vi "Man Simulation V2.vi"() -> ()   [LabVIEW 2020]
panel:
  out "J in 1 NS pair with gap":dbl
  out "Energy (wh/m3) / 1 NS pari with gap":dbl
  out "Energy Density  WH/m3":dbl
  in  "Energy Density  WH/Lit":dbl
  out "1 NS Pair Energy / Volume":dbl
  out "1 NS Pair Energy / mass":dbl
  out "Chip Energy Wh":dbl
  out "WH/Lit":dbl
  out "WH/m3":dbl
  out "WH/Kg":dbl
  out "Chip Energy / Volume":dbl
  out "Chip Energy /Mass":dbl
  out "Mass of a Chip":dbl
  out "Volume of a Chip":dbl
  out "Mass NS Pair with Gap":dbl
  out "Volume NS Pair With Gap":dbl
  out "Volume Gap":dbl
  out "Mass Gap":dbl
  out "Delta Temp Change \nDielectric Gap":dbl
  out "Dielectric Thickness  \nGap":dbl
  out "Mass Dielectric \nGap":dbl
  out "Volume Dielectric \nGap":dbl
  out "Delta Temp Change\n SiO2 Gap":dbl
  out "Mass SiO2 Gap":dbl
  out "Sio2 Thickness Gap":dbl
  out "Volume SiO2 Gap":dbl
  out "Volume Si Gap":dbl
  out "Silicon Thickness Gap":dbl
  out "Mass Si Gap":dbl
  out "Delta Temp Change\n Si Gap":dbl
  out "Area B/W NS":dbl
  out "Vol 2 NS":dbl
  out "Mass 2 NS":dbl
  out "Mass 1 NS":dbl
  out "Volume 1 NS":dbl
  out "SiO2 Specfic Heat Capacity 2":dbl
  out "SilO2 Density 2":dbl
  out "Delta Temp Change SiO2 2":dbl
  out "Mass SiO2 2":dbl
  out "Volume SiO2 2":dbl
  out "Dielectric Specfic Heat Capacity":dbl
  out "Dielectric Density":dbl
  out "CNT Specfic Heat Capacity":dbl
  out "CNT Density":dbl
  out "Fe Specfic Heat Capacity":dbl
  out "Fe Density":dbl
  out "Al Specfic Heat Capacity":dbl
  out "Al Density":dbl
  out "Al2O3 Specfic Heat Capacity":dbl
  out "Al2O3 Density":dbl
  out "M1 Specfic Heat Capacity":dbl
  out "M1 Density":dbl
  out "SiO2 Specfic Heat Capacity":dbl
  out "SilO2 Density":dbl
  out "um in 1 inch":dbl
  out "Microns":dbl
  in  "Inches":dbl
  in  "Energy (Heat; I^2R)":dbl
  out "Delta Temp Change \nDielectric":dbl
  out "Mass Dielectric":dbl
  out "Volume Dielectric":dbl
  out "Delta Temp Change CNT":dbl
  out "Mass CNTs":dbl
  out "Volume CNT":dbl
  out "Delta Temp Change Fe":dbl
  out "Mass Fe":dbl
  out "Volume Fe":dbl
  out "Delta Temp Change Al":dbl
  out "Mass  Al":dbl
  out "Volume Al":dbl
  out "Delta Temp Change Al2O3":dbl
  out "Mass Al2O3":dbl
  out "Volume Al2O3":dbl
  out "Delta Temp Change M1":dbl
  out "Mass M1":dbl
  out "Volume M1":dbl
  out "Delta Temp Change SiO2":dbl
  out "Mass SiO2":dbl
  out "Volume SiO2":dbl
  out "Dielectric Thickness":dbl
  out "CNT Thickness":dbl
  out "Fe Thickness":dbl
  out "Al Thickness":dbl
  out "Al2O3 Thickness":dbl
  out "M1 Thickness":dbl
  out "SiO2 Thickness 2":dbl
  out "Sio2 Thickness":dbl
  out "Silicon Thickness":dbl
  out "m-nm Dielectric":dbl
  out "Dielectric Thickness":dbl
  out "m-nm CNT":dbl
  out "CNT Thickness (CNT Length)":dbl
  in  "m-nm Fe":dbl
  in  "Fe Thickness":dbl
  in  "m-nm Al":dbl
  in  "Aluminum Thickness":dbl
  out "Heat Generated (Energy) by Current in Metal films":dbl
  out "Delta Temp Change Si":dbl
  out "Silicon Specfic Heat Capacity":dbl
  out "Silicon Density":dbl
  out "Mass Si":dbl
  out "Volume Si":dbl
  in  "m-nm SiO2 2":dbl
  in  "Silicon DiOxide Thickness  2":dbl
  in  "m-nm Al2O3":dbl
  in  "m-nm M1":dbl
  in  "Alumina Thickness":dbl
  in  "Metal 1 (Ti)":dbl
  in  "m-nm SiO2":dbl
  in  "m-nm Si":dbl
  in  "Silicon DiOxide Thickness":dbl
  in  "Silicon Thickness":dbl
  out "Rf for Max i;  R+ C (EDL+Funct)":dbl
  out "Rf for Max i;  R+ C (EDL+Funct+ Analyte)":dbl
  in  "Max V_out":dbl
  out "Delta i":dbl
  out "Max i;  R+ C (EDL+Funct+ Analyte)":dbl format="%#_9e"
  out "Max i;  R+ C (EDL+Funct)":dbl format="%#_9e"
  out "V_Zeta":dbl
  out "|Z| of R+ C (EDL+Funct+Analyte)":dbl
  out "|Z| of R+ C (EDL+Funct)":dbl
  out "Delta Total Impedance":dbl
  out "Total Impedance Rs+C(EDS+Funct+Analyte)":dbl
  out "Total Impedance Rs+C(EDS+Funct)":dbl
  in  "Series Resistance of Solution":dbl
  in  "Freq Hz-MHz":dbl
  out "Impedance of EDL & Functionalization & Analyte":dbl
  out "Impedance of EDL & Functionalization":dbl
  in  "Frequency":dbl
  out "Delta C":dbl
  out "Capacitance of ELD & Functionalization & Analyte":dbl
  out "Capacitance of ELD & Functionalization":dbl
  out "C_EDL/ 1 NS":dbl
  out "C_EDL/ 1 CNT":dbl
  out "C EDL by d with Cosh Factor":dbl format="%#_6e"
  out "C EDL by d":dbl
  out "d; EDL Length":dbl
  out "R=kN_a":dbl
  out "F=eN_a":dbl
  out "N_a; Avagadro no":dbl=1.38064852e-23
  in  "V  nV-m V-V":dbl
  out "C_EDL/ A":dbl format="%#_6e"
  out "c; Charge on e":dbl=1.6021766208e-19
  in  "V zeta":dbl
  out "C in M":dbl
  in  "Co nM-M":dbl
  in  "T":dbl
  out "k; Boltzmann Constant":dbl=1.38064852e-23
  in  "Co; miliMolar (moles/m3)":dbl
  in  "er":dbl
  out "eo; Permitivity of Free Space":dbl=8.85418782e-12
  in  "z":dbl
  out "Length of CNTs  2":dbl
  in  "Dielectric of Molecule 2 Analyte":dbl
  out "Capacitance Functinal Analyte  per unit area":dbl
  out "Capaciatance per CNT Analyte":dbl
  out "Capacitance Functional Analyte per NS":dbl
  out "Capacitance Functional Analyte per NS 2":dbl
  out "Gap B/w NS":dbl
  out "Chip Impedance":dbl
  out "Chip Capacitance":dbl
  out "Chip Energy":dbl
  out "Chip Power":dbl
  in  "Freq Hz K; M Hz":dbl
  out "Power":dbl
  in  "Frequency":dbl
  out "Impedance":dbl
  in  "Voltage":dbl
  out "Energy":dbl
  out "Capacitance of 1 Pair NS":dbl(graph)
  out "Capacitance of 1 Pair NS":dbl
  in  "er":dbl
  out "Capacitance Functional Molecules per NS 2":dbl
  out "Capacitance Functional Molecules per NS":dbl
  out "Capaciatance per CNT Functional":dbl
  out "Capacitance Functinal Molecule  per unit area":dbl
  in  "Dielectric of Molecule":dbl
  out "Concentration,  M":ext[unit]
  out "Concentration on 1 NS (Moles/m3)":ext[unit]
  out "Total Functionalized Molecules on NS":dbl
  out "No of Molecules on 1 CNT Functionalized":dbl
  out "Molecule Length Analyte":dbl
  out "Molecle Area with Gap Analyte":dbl
  out "Volume of Molecule Analyte":dbl
  out "Area of Molecule on CNT surface Analyte":dbl
  in  "m-nm Gap Molecules Analyte":dbl caption="m-nm Gap"
  in  "Gap Between Molecules Analyte":dbl caption="Gap Between CNTs"
  in  "m-nm l Molecule Analyte":dbl
  in  "m-nm r Molecule Analyte":dbl caption="m-nm r"
  in  "Length of Molecule Analyte":dbl caption="Length of CNTs"
  in  "Radius of Molecule Analyte":dbl caption="Radius of CNTs"
  out "Molecule Length":dbl
  out "Molecle Area with Gap":dbl
  out "Volume of Molecule":dbl
  out "Area of Molecule on CNT surface":dbl
  in  "m-nm Gap Molecules":dbl caption="m-nm Gap"
  in  "Gap Between Molecules":dbl caption="Gap Between CNTs"
  in  "m-nm l Molecule":dbl
  in  "m-nm r Molecule":dbl caption="m-nm r"
  in  "Length of Molecule":dbl caption="Length of CNTs"
  in  "Radius of Molecule":dbl caption="Radius of CNTs"
  out "NS Width":dbl
  out "No of NS Pairs on Chip":dbl
  in  "Gap n-m":dbl
  in  "Gap B/W NS":dbl
  in  "m-nm LChip":dbl
  in  "m-nm WChip":dbl
  in  "Length of Chip":dbl
  in  "Width of Chip":dbl
  out "Surface Area 1 NS":dbl
  out "# of CNTs in 1 NS":dbl format="%#_6e"
  out "Area 1 CNT & Gap":dbl
  out "NS Length":dbl
  out "NS Base Area":dbl
  out "CNT Radius":dbl
  out "CNT Base Area":dbl
  out "XY Graph":cluster{"X":dbl[], "Y":dbl[]}[](graph)
  in  "m-nm NS Base":dbl caption="m-nm 4"
  in  "m-nm WB":dbl
  in  "Length of Base":dbl
  in  "Width of Base":dbl
  in  "m-nm Gap":dbl
  in  "Gap Between CNTs":dbl
  out "Surface Area of 1 CNT":dbl
  in  "m-nm l":dbl
  in  "m-nm r":dbl
  in  "Length of CNTs":dbl
  in  "Radius of CNTs":dbl
  # "CAP"
  # "Chip CAP"
  # "Chip NanoStructure"
  # "CNT Nanostructure"
  # "CAP Design"
  # "Nano Structure Material Stack"
  # "Constants for Materials in Stack"
  # "Nano Structure"
  # "Chip"
  # "Dielectric =1/2 of Gap B/w NS"
  # "Analyte Molecule"
  # "Functionalization Molecule"
  # "Analyte Attached to Functionalized  NanoStructure"
  # "TiO2: 4260 kg/m3\nHafnium Odide: 9680"
  # "GAP B/W NS  Material"
  # "Capacitance of Analyte Molecule on NanoStructure"
  # "Functionalized NanoStructure"
  # "Mass and Volume of NS Pair"
  # "Molecule Fnctionalization"
  # "Capacitance of Functional Molecule on NanoStructure"
  # "Mass and Volume of Chip"
  # "Echem & Electrical Signals"
  # "Electric Double Layer; EDL"
  # "Constants"
  # "Cosh(zeV_zeta/2kT)"
  # "Potentiostat"
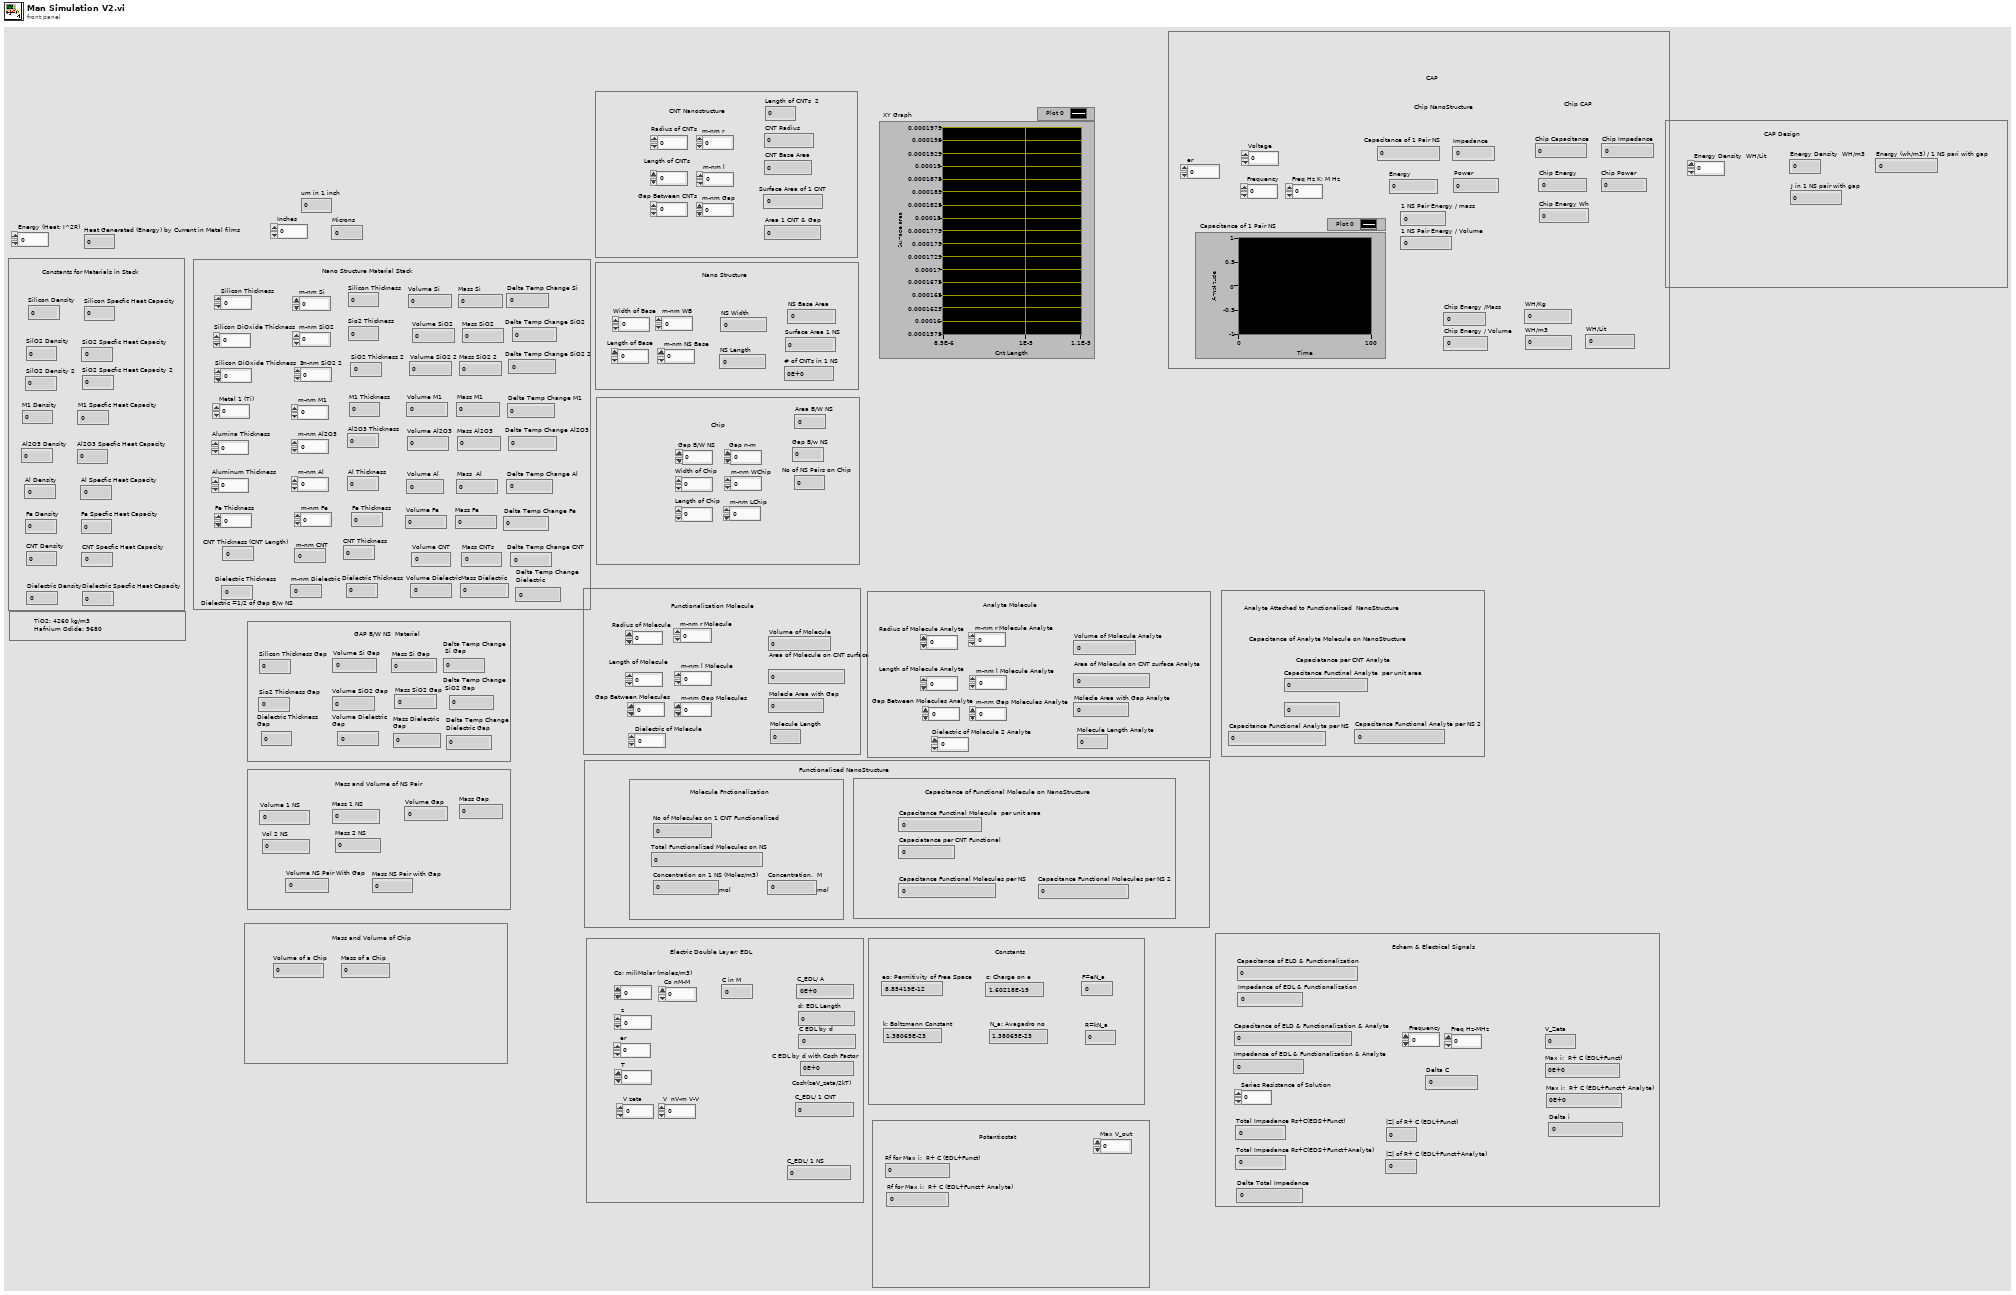
[diagram p1: front panel]
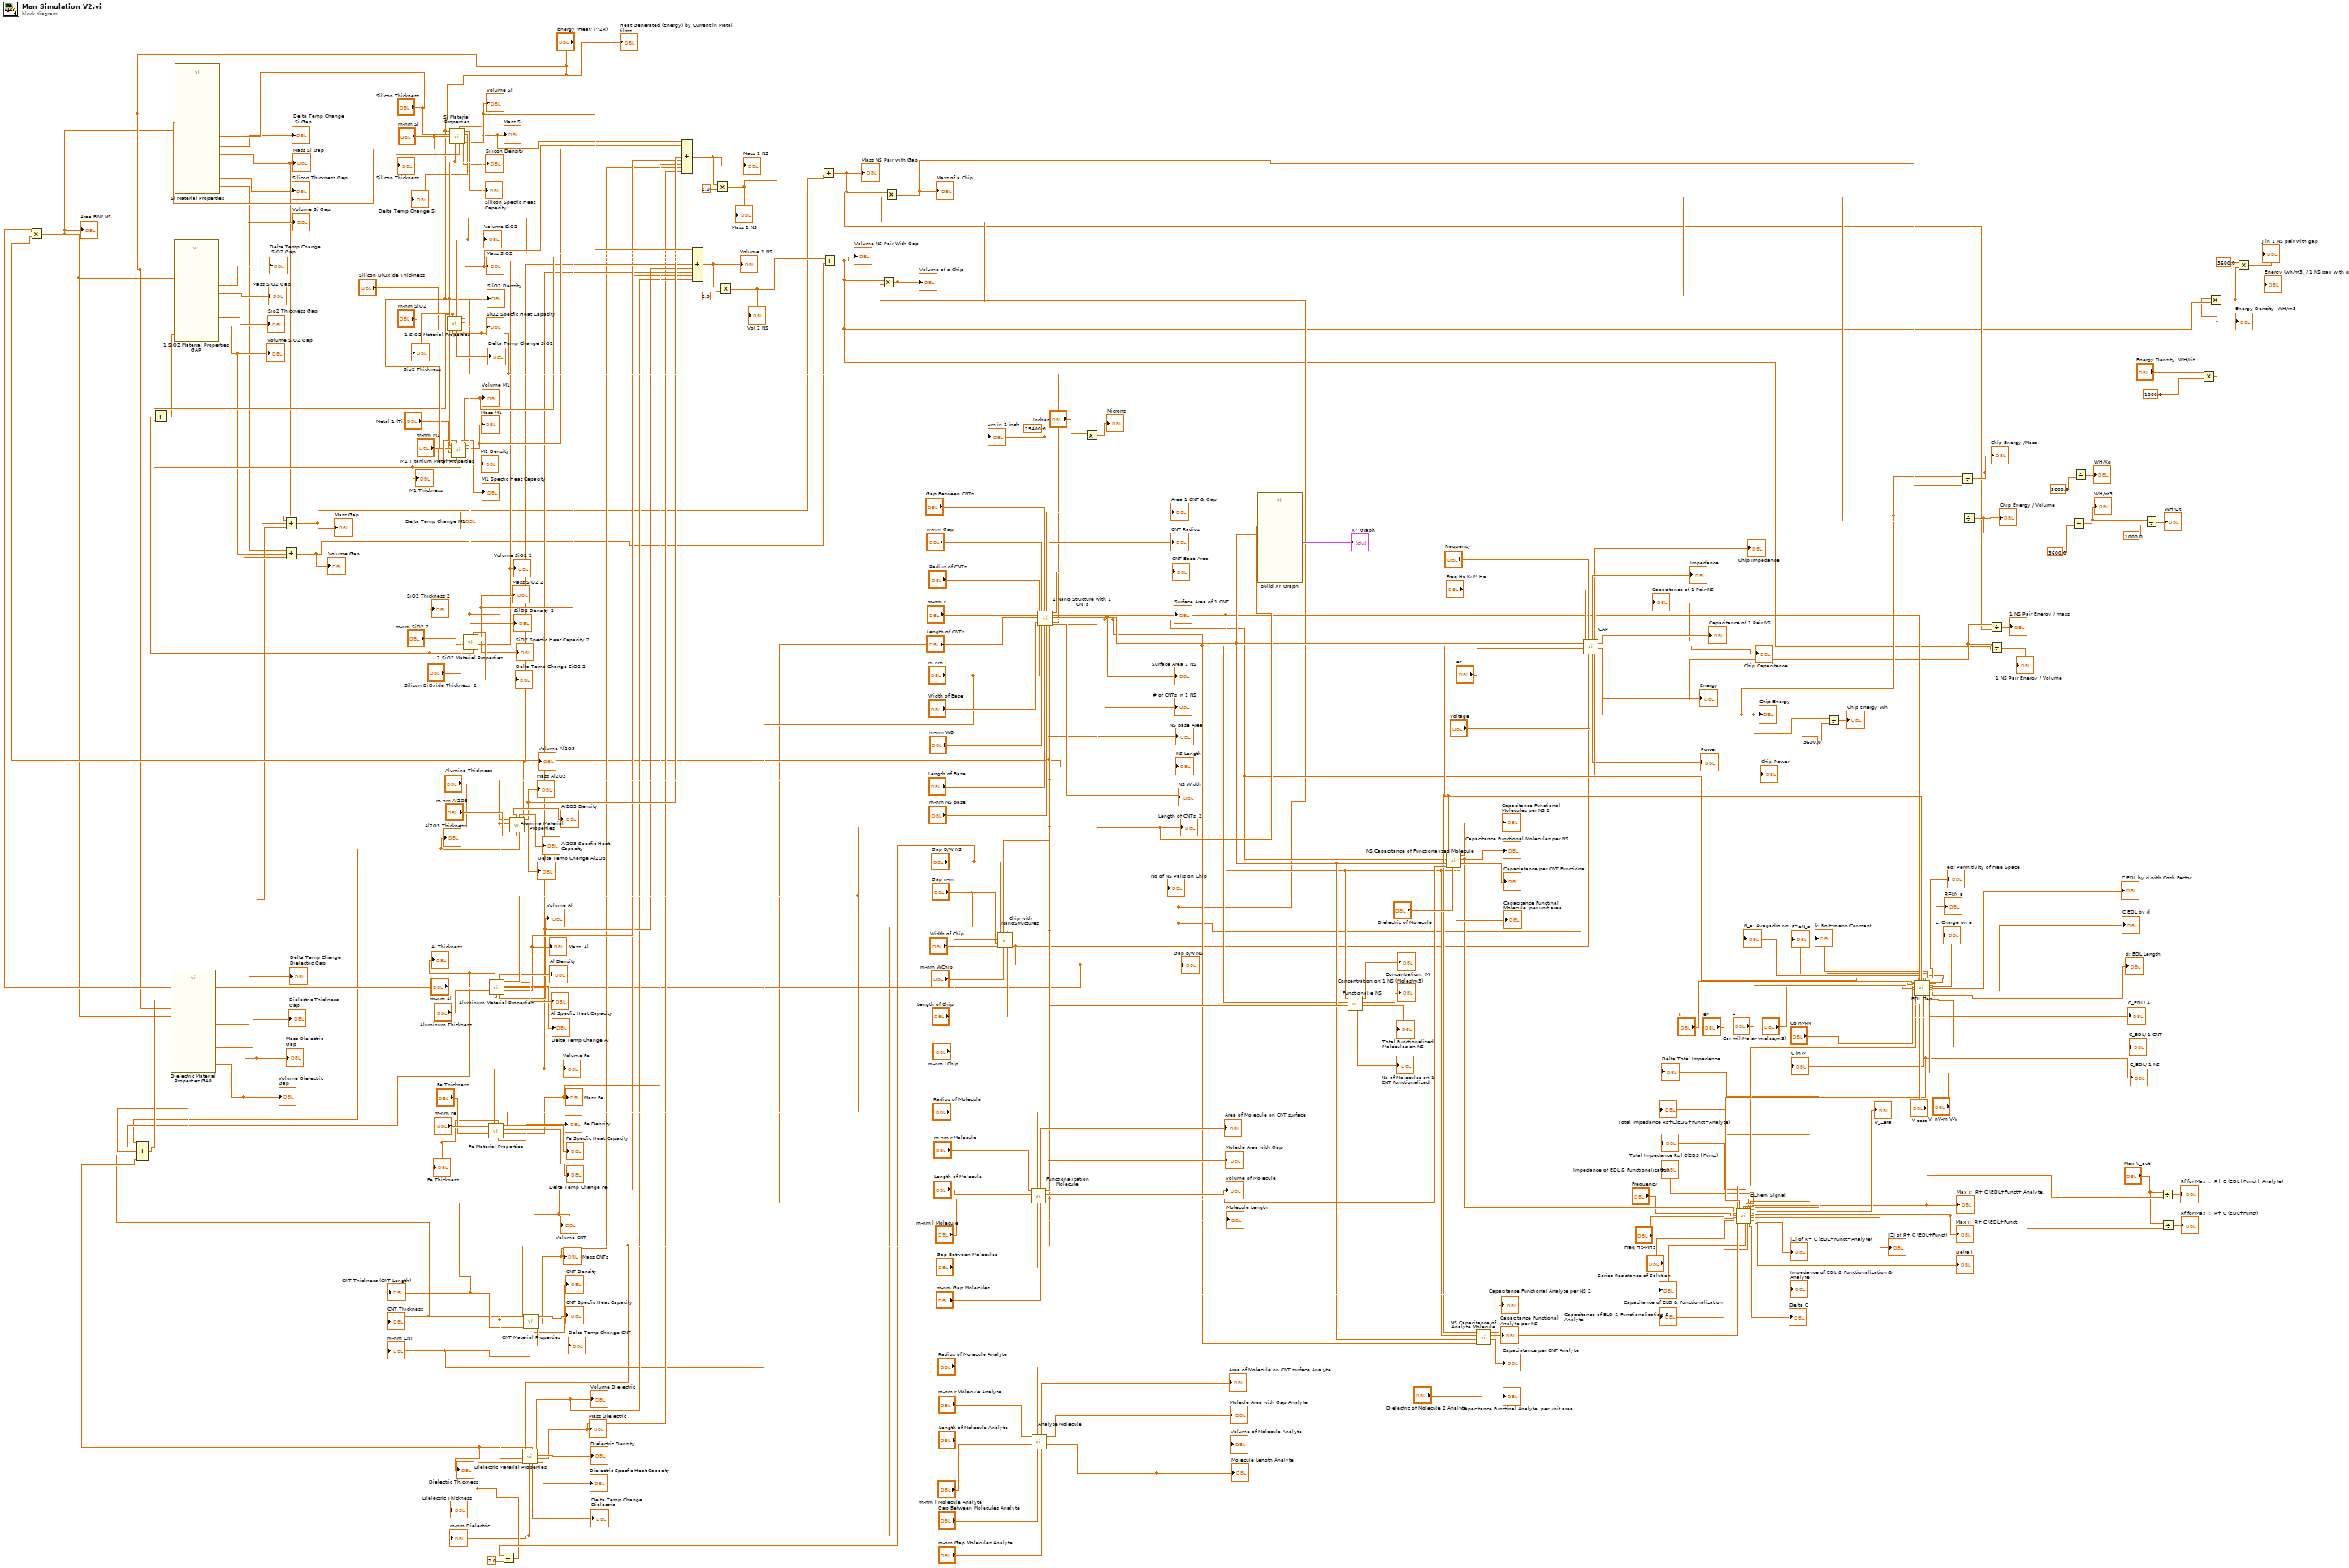
[diagram p0: block diagram]
diagram:
  w102 = 25400.0 ("y")
  n1 = Divide(x="Gap B/W NS", y=2.0) -> (x/y=w53:dbl)
  "Dielectric Thickness" <- w53
  n2 = call "Functionalization Molecule.vi"("m-nm Gap Molecules"="m-nm Gap Molecules", "Gap Between Molecules"="Gap Between Molecules", "Radius of Molecule"="Radius of Molecule", "m-nm l Molecule"="m-nm l Molecule", "Length of Molecule"="Length of Molecule", "m-nm r Molecule"="m-nm r Molecule") -> ("Molecule Length"=w197:dbl, "Volume of Molecule"=→"Volume of Molecule":dbl, "Molecle Area with Gap"=w203:dbl, "Area of Molecule on CNT surface"=→"Area of Molecule on CNT surface":dbl)  [unwired: 2 in]
  "Molecle Area with Gap" <- w203
  "Molecule Length" <- w197
  n3 = call "Analyte Molecule.vi"("m-nm Gap Molecules"="m-nm Gap Molecules Analyte", "Gap Between Molecules"="Gap Between Molecules Analyte", "Radius of Molecule"="Radius of Molecule Analyte", "m-nm l Molecule"="m-nm l Molecule Analyte", "Length of Molecule"="Length of Molecule Analyte", "m-nm r Molecule"="m-nm r Molecule Analyte") -> ("Molecule Length"=w181:dbl, "Volume of Molecule"=→"Volume of Molecule Analyte":dbl, "Molecle Area with Gap"=→"Molecle Area with Gap Analyte":dbl, "Area of Molecule on CNT surface"=→"Area of Molecule on CNT surface Analyte":dbl)  [unwired: 2 in]
  "Molecule Length Analyte" <- w181
  n4 = call "1 Nano Structure with 1 CNTs.vi"("Radius of CNTs"="Radius of CNTs", "m-nm r"="m-nm r", "Length of CNTs"="Length of CNTs", "m-nm l"="m-nm l", "Width of Base"="Width of Base", "m-nm Gap"="m-nm Gap", "m-nm WB"="m-nm WB", "Gap Between CNTs"="Gap Between CNTs", "Length of Base"="Length of Base", "m-nm NS Base"="m-nm NS Base") -> ("Length of CNTs"=w178:dbl, "Area 1 CNT & Gap"=→"Area 1 CNT & Gap":dbl, "CNT Radius"=→"CNT Radius":dbl, "NS Length"=w68:dbl, "CNT Base Area"=→"CNT Base Area":dbl, "Surface Area of 1 CNT"=w168:dbl, "Surface Area 1 NS"=w177:dbl, "# of CNTs in 1 NS"=w167:dbl, "NS Base Area"=w125:dbl, "NS Width"=→"NS Width":dbl)
  "Surface Area of 1 CNT" <- w168
  "NS Base Area" <- w125
  "NS Length" <- w68
  "# of CNTs in 1 NS" <- w167
  "Surface Area 1 NS" <- w177
  "Length of CNTs  2" <- w178
  n5 = call "1 SiO2 Material Properties.vi"("NS Base Area"=w125, "Silicon DiOxide Thickness  in"="Silicon DiOxide Thickness", "m-nm SiO2 in"="m-nm SiO2", "Energy (Heat; I^2R)"="Energy (Heat; I^2R)") -> ("SiO2 Specfic Heat Capacity"=→"SiO2 Specfic Heat Capacity":dbl, "Mass SiO2"=w93:dbl, "SilO2 Density"=→"SilO2 Density":dbl, "Delta Temp Change SiO2"=→"Delta Temp Change SiO2":dbl, "Volume SiO2"=w92:dbl, "Sio2 Thickness"=w41:dbl)  [unwired: 1 in, 1 out]
  "Sio2 Thickness" <- w41
  "Volume SiO2" <- w92
  "Mass SiO2" <- w93
  n6 = call "Si Material Properties.vi"("NS Base Area"=w125, "m-nm Si"="m-nm Si", "Silicon Thickness in"="Silicon Thickness", "Energy (Heat; I^2R)"="Energy (Heat; I^2R)") -> ("Volume Si"=w95:dbl, "Silicon Density"=→"Silicon Density":dbl, "Delta Temp Change Si"=→"Delta Temp Change Si":dbl, "Silicon Specfic Heat Capacity"=→"Silicon Specfic Heat Capacity":dbl, "Silicon Thickness out"=→"Silicon Thickness":dbl, "Mass Si"=w94:dbl)  [unwired: 1 in, 1 out]
  "Volume Si" <- w95
  "Mass Si" <- w94
  n7 = call "M1 Titanium Metal Properties.vi"("m-nm M1"="m-nm M1", "Metal 1 (Ti)"="Metal 1 (Ti)", "Energy (Heat; I^2R)"="Energy (Heat; I^2R)", "NS Base Area"=w125) -> ("Volume M1"=w90:dbl, "Mass M1"=w91:dbl, "Delta Temp Change M1"=→"Delta Temp Change M1":dbl, "M1 Thickness"=w43:dbl, "M1 Specfic Heat Capacity"=→"M1 Specfic Heat Capacity":dbl, "M1 Density"=→"M1 Density":dbl)  [unwired: 1 in, 1 out]
  "M1 Thickness" <- w43
  "Volume M1" <- w90
  "Mass M1" <- w91
  n8 = call "2 SiO2 Material Properties.vi"("NS Base Area"=w125, "m-nm SiO2 in"="m-nm SiO2 2", "Silicon DiOxide Thickness  in"="Silicon DiOxide Thickness  2", "Energy (Heat; I^2R)"="Energy (Heat; I^2R)") -> ("Volume SiO2 2"=w88:dbl, "SiO2 Specfic Heat Capacity 2"=→"SiO2 Specfic Heat Capacity 2":dbl, "Mass SiO2 2"=w89:dbl, "SiO2 Thickness 2"=w42:dbl, "Delta Temp Change SiO2 2"=→"Delta Temp Change SiO2 2":dbl, "SilO2 Density 2"=→"SilO2 Density 2":dbl)  [unwired: 1 in, 1 out]
  "SiO2 Thickness 2" <- w42
  "Volume SiO2 2" <- w88
  "Mass SiO2 2" <- w89
  n9 = Compound Arithmetic op=ADD(w41, w42, w43) -> (w40:dbl)
  n10 = call "Fe Material Properties.vi"("m-nm Fe"="m-nm Fe", "Fe Thickness"="Fe Thickness", "Energy (Heat; I^2R)"="Energy (Heat; I^2R)", "NS Base Area"=w125) -> ("Mass Fe"=w82:dbl, "Delta Temp Change Fe"=→"Delta Temp Change Fe":dbl, "Fe Specfic Heat Capacity"=→"Fe Specfic Heat Capacity":dbl, "Fe Density"=→"Fe Density":dbl, "Fe Thickness 2"=w48:dbl, "Volume Fe"=w83:dbl)  [unwired: 1 in, 1 out]
  "Fe Thickness" <- w48
  "Volume Fe" <- w83
  "Mass Fe" <- w82
  n11 = call "Aluminum Material Properties.vi"("m-nm Al"="m-nm Al", "Aluminum Thickness"="Aluminum Thickness", "Energy (Heat; I^2R)"="Energy (Heat; I^2R)", "NS Base Area"=w125) -> ("Mass  Al"=w85:dbl, "Delta Temp Change Al"=→"Delta Temp Change Al":dbl, "Al Specfic Heat Capacity"=→"Al Specfic Heat Capacity":dbl, "Volume Al"=w84:dbl, "Al Density"=→"Al Density":dbl, "Al Thickness"=w45:dbl)  [unwired: 1 in, 1 out]
  "Al Thickness" <- w45
  "Volume Al" <- w84
  "Mass  Al" <- w85
  n12 = call "Alumina Material Properties.vi"("m-nm Al2O3"="m-nm Al2O3", "Alumina Thickness"="Alumina Thickness", "Energy (Heat; I^2R)"="Energy (Heat; I^2R)", "NS Base Area"=w125) -> ("Volume Al2O3"=w86:dbl, "Delta Temp Change Al2O3"=→"Delta Temp Change Al2O3":dbl, "Mass Al2O3"=w87:dbl, "Al2O3 Thickness"=w44:dbl, "Al2O3 Specfic Heat Capacity"=→"Al2O3 Specfic Heat Capacity":dbl, "Al2O3 Density"=→"Al2O3 Density":dbl)  [unwired: 1 in, 1 out]
  "Al2O3 Thickness" <- w44
  "Volume Al2O3" <- w86
  "Mass Al2O3" <- w87
  n13 = call "Dielectric Material Properties.vi"("m-nm Dielectric"="Gap n-m", "Dielectric Thickness  in"=w53, "Energy (Heat; I^2R)"="Energy (Heat; I^2R)", "NS Base Area"=w125) -> ("Dielectric Specfic Heat Capacity"=→"Dielectric Specfic Heat Capacity":dbl, "Mass Dielectric"=w78:dbl, "Dielectric Density"=→"Dielectric Density":dbl, "Volume Dielectric"=w79:dbl, "Delta Temp Change \nDielectric"=→"Delta Temp Change \nDielectric":dbl, "Dielectric Thickness  out"=w47:dbl)  [unwired: 1 in, 1 out]
  "Dielectric Thickness" <- w47
  "Volume Dielectric" <- w79
  "Mass Dielectric" <- w78
  n14 = call "CNT Material Properties.vi"("m-nm CNT"="m-nm l", "CNT Thickness (CNT Length)"="Length of CNTs", "Energy (Heat; I^2R)"="Energy (Heat; I^2R)", "NS Base Area"=w125) -> ("Mass CNTs"=w81:dbl, "Delta Temp Change CNT"=→"Delta Temp Change CNT":dbl, "CNT Specfic Heat Capacity"=→"CNT Specfic Heat Capacity":dbl, "CNT Density"=→"CNT Density":dbl, "Volume CNT"=w80:dbl, "CNT Thickness"=w46:dbl)  [unwired: 1 in, 1 out]
  "CNT Thickness" <- w46
  "Volume CNT" <- w80
  "Mass CNTs" <- w81
  n15 = Compound Arithmetic op=ADD(w44, w45, w48, w46, w47) -> (w54:dbl)
  n16 = Compound Arithmetic op=ADD(w94, w93, w91, w89, w87, w85, w82, w81, w78) -> (w75:dbl)
  "Mass 1 NS" <- w75
  n17 = Compound Arithmetic op=ADD(w95, w92, w90, w88, w86, w84, w83, w80, w79) -> (w74:dbl)
  "Volume 1 NS" <- w74
  n18 = Multiply(x=w75, y=2.0) -> (x*y=w30:dbl)
  "Mass 2 NS" <- w30
  n19 = Multiply(x=w74, y=2.0) -> (x*y=w29:dbl)
  "Vol 2 NS" <- w29
  n20 = call "Chip with NanoStructures.vi"("Length of Chip"="Length of Chip", "NS Base Area"=w125, "m-nm WChip"="m-nm WChip", "NS Length"=w68, "Width of Chip"="Width of Chip", "Gap n-m"="Gap n-m", "m-nm LChip"="m-nm LChip", "Gap B/W NS"="Gap B/W NS") -> ("Gap B/w NS"=w67:dbl, "No of NS Pairs on Chip"=w26:dbl)  [unwired: 2 in]
  "No of NS Pairs on Chip" <- w26
  "Gap B/w NS" <- w67
  n21 = Multiply(x=w67, y=w68) -> (x*y=w59:dbl)
  "Area B/W NS" <- w59
  n22 = call "Dielectric Material Properties GAP.vi"("Dielectric Thickness Total"=w54, "Energy (Heat; I^2R)"="Energy (Heat; I^2R)", "NS Base Area"=w59) -> ("Mass Dielectric"=w31:dbl, "Volume Dielectric"=w32:dbl, "Delta Temp Change \nDielectric"=→"Delta Temp Change \nDielectric Gap":dbl, "Dielectric Thickness  out"=→"Dielectric Thickness  \nGap":dbl)  [unwired: 3 in, 2 out]
  "Volume Dielectric \nGap" <- w32
  "Mass Dielectric \nGap" <- w31
  n23 = call "1 SiO2 Material Properties GAP.vi"("NS Base Area"=w59, "Sio2 Thickness 2"=w40, "Energy (Heat; I^2R)"="Energy (Heat; I^2R)") -> ("Mass SiO2"=w35:dbl, "Delta Temp Change SiO2"=→"Delta Temp Change\n SiO2 Gap":dbl, "Volume SiO2"=w36:dbl, "Sio2 Thickness"=→"Sio2 Thickness Gap":dbl)  [unwired: 3 in, 2 out]
  "Volume SiO2 Gap" <- w36
  "Mass SiO2 Gap" <- w35
  n24 = call "Si Material Properties.vi"("NS Base Area"=w59, "m-nm Si"="m-nm Si", "Silicon Thickness in"="Silicon Thickness", "Energy (Heat; I^2R)"="Energy (Heat; I^2R)") -> ("Volume Si"=w34:dbl, "Delta Temp Change Si"=→"Delta Temp Change\n Si Gap":dbl, "Silicon Thickness out"=→"Silicon Thickness Gap":dbl, "Mass Si"=w33:dbl)  [unwired: 1 in, 3 out]
  "Mass Si Gap" <- w33
  "Volume Si Gap" <- w34
  n25 = Compound Arithmetic op=ADD(w33, w35, w31) -> (w28:dbl)
  "Mass Gap" <- w28
  n26 = Compound Arithmetic op=ADD(w34, w36, w32) -> (w27:dbl)
  "Volume Gap" <- w27
  n27 = Add(x=w30, y=w28) -> (x+y=w8:dbl)
  "Mass NS Pair with Gap" <- w8
  n28 = Add(x=w29, y=w27) -> (x+y=w5:dbl)
  "Volume NS Pair With Gap" <- w5
  n29 = Multiply(x=w5, y=w26) -> (x*y=w24:dbl)
  "Volume of a Chip" <- w24
  n30 = Multiply(x=w8, y=w26) -> (x*y=w25:dbl)
  "Mass of a Chip" <- w25
  n31 = Multiply(x="Inches", y=w102) -> (x*y=→"Microns":dbl)
  n32 = call "Build XY Graph"("Y Input"=w177, "X Input"=w178) -> ("XY Graph"=→"XY Graph":cluster{"X":dbl[], "Y":dbl[]}[])  [unwired: 8 in, 1 out]
  n33 = call "Functionalie NS.vi"("Molecle Area with Gap"=w203, "# of CNTs in 1 NS"=w167, "Surface Area of 1 CNT"=w168) -> ("Total Functionalized Molecules on NS"=→"Total Functionalized Molecules on NS":dbl, "Concentration on 1 NS (Moles/m3)"=→"Concentration on 1 NS (Moles/m3)":ext[unit], "Concentration,  M"=→"Concentration,  M":ext[unit], "No of Molecules on 1 CNT Functionalized"=→"No of Molecules on 1 CNT Functionalized":dbl)  [unwired: 5 in]
  n34 = call "EDL Cap.vi"("T"="T", "er"="er", "z"="z", "Co; miliMolar (moles/m3)"="Co; miliMolar (moles/m3)", "Co nM-M"="Co nM-M", "V  nV-m V-V"="V  nV-m V-V", "V zeta"="V zeta", "# of CNTs in 1 NS"=w167, "Surface Area of 1 CNT"=w168) -> ("V_Zeta"=w147:dbl, "eo; Permitivity of Free Space 2"=w169:dbl, "N_a; Avagadro no"=→"N_a; Avagadro no":dbl, "C in M"=→"C in M":dbl, "eo; Permitivity of Free Space"=→"eo; Permitivity of Free Space":dbl, "C_EDL/ 1 NS"=w152:dbl, "k; Boltzmann Constant"=→"k; Boltzmann Constant":dbl, "C_EDL/ 1 CNT"=→"C_EDL/ 1 CNT":dbl, "F=eN_a"=→"F=eN_a":dbl, "R=kN_a"=→"R=kN_a":dbl, "c; Charge on e"=→"c; Charge on e":dbl, "C EDL by d with Cosh Factor"=→"C EDL by d with Cosh Factor":dbl, "C EDL by d"=→"C EDL by d":dbl, "d; EDL Length"=→"d; EDL Length":dbl, "C_EDL/ A"=→"C_EDL/ A":dbl)  [unwired: 4 in]
  "C_EDL/ 1 NS" <- w152
  n35 = call "NS Capacitance of Functionalized Molecule.vi"("SA of 1 CNT"=w168, "Dielectric of Molecule"="Dielectric of Molecule", "Molecule Length"=w197, "Surface Area 1 NS"=w177, "# of CNTs"=w167, "Permitivity of Free Space"=w169) -> ("Capaciatance per CNT"=→"Capaciatance per CNT Functional":dbl, "Capacitance Functional Molecules per NS"=w153:dbl, "Capacitance Functional Molecules per NS 2"=→"Capacitance Functional Molecules per NS 2":dbl, "Capacitance Functinal Molecule  per unit area"=→"Capacitance Functinal Molecule  per unit area":dbl)  [unwired: 2 in]
  "Capacitance Functional Molecules per NS" <- w153
  n36 = call "NS Capacitance of Analyte Molecule.vi"("Dielectric of Molecule Analyte"="Dielectric of Molecule 2 Analyte", "Molecule Length"=w181, "# of CNTs"=w167, "Surface Area 1 NS"=w177, "Surface Area of 1 CNT"=w168, "Permitivity of Free Space"=w169) -> ("Capaciatance per CNT"=→"Capaciatance per CNT Analyte":dbl, "Capacitance Functional Analyte per NS"=w154:dbl, "Capacitance Functional Analyte per NS 2"=→"Capacitance Functional Analyte per NS 2":dbl, "Capacitance Functinal Analyte  per unit area"=→"Capacitance Functinal Analyte  per unit area":dbl)  [unwired: 2 in]
  "Capacitance Functional Analyte per NS" <- w154
  n37 = call "CAP.vi"("Freq Hz K; M Hz"="Freq Hz K; M Hz", "Surface Area 1 NS"=w177, "Permitivity of Free Space"=w169, "er"="er", "No of NS Pairs on Chip"=w26, "Frequency"="Frequency", "Gap B/w NS"=w67, "Voltage"="Voltage") -> ("Impedance"=→"Impedance":dbl, "Power"=→"Power":dbl, "Chip Impedance"=→"Chip Impedance":dbl, "Chip Power"=→"Chip Power":dbl, "Capacitance of 1 Pair NS"=→"Capacitance of 1 Pair NS":dbl, "Capacitance of 1 Pair"=→"Capacitance of 1 Pair NS":dbl, "Chip Capacitance"=→"Chip Capacitance":dbl, "Chip Energy"=w14:dbl, "Energy"=w9:dbl)  [unwired: 3 in]
  "Energy" <- w9
  "Chip Energy" <- w14
  n38 = call "EChem Signal.vi"("V_Zeta in"=w147, "Capacitance Functional Molecules per NS"=w153, "Series Resistance of Solution"="Series Resistance of Solution", "Frequency"="Frequency", "Freq Hz-MHz"="Freq Hz-MHz", "Capacitance Functional Analyte per NS"=w154, "C_EDL/ 1 NS"=w152) -> ("Impedance of EDL & Functionalization & Analyte"=→"Impedance of EDL & Functionalization & Analyte":dbl, "Impedance of EDL & Functionalization"=→"Impedance of EDL & Functionalization":dbl, "Capacitance of ELD & Functionalization"=→"Capacitance of ELD & Functionalization":dbl, "Total Impedance Rs+C(EDS+Funct)"=→"Total Impedance Rs+C(EDS+Funct)":dbl, "Capacitance of ELD & Functionalization & Analyte"=→"Capacitance of ELD & Functionalization & Analyte":dbl, "Total Impedance Rs+C(EDS+Funct+Analyte)"=→"Total Impedance Rs+C(EDS+Funct+Analyte)":dbl, "Delta C"=→"Delta C":dbl, "Delta Total Impedance"=→"Delta Total Impedance":dbl, "V_Zeta out"=→"V_Zeta":dbl, "Max i;  R+ C (EDL+Funct)"=w131:dbl, "|Z| of R+ C (EDL+Funct)"=→"|Z| of R+ C (EDL+Funct)":dbl, "Delta i"=→"Delta i":dbl, "Max i;  R+ C (EDL+Funct+ Analyte)"=w135:dbl, "|Z| of R+ C (EDL+Funct+Analyte)"=→"|Z| of R+ C (EDL+Funct+Analyte)":dbl)  [unwired: 7 in]
  "Max i;  R+ C (EDL+Funct)" <- w131
  "Max i;  R+ C (EDL+Funct+ Analyte)" <- w135
  n39 = Divide(x=w14, y=3600.0) -> (x/y=→"Chip Energy Wh":dbl)
  n40 = Divide(x=w14, y=w25) -> (x/y=w22:dbl)
  "Chip Energy /Mass" <- w22
  n41 = Divide(x=w14, y=w24) -> (x/y=w19:dbl)
  "Chip Energy / Volume" <- w19
  n42 = Divide(x=w9, y=w8) -> (x/y=→"1 NS Pair Energy / mass":dbl)
  n43 = Divide(x=w9, y=w5) -> (x/y=→"1 NS Pair Energy / Volume":dbl)
  n44 = Divide(x=w19, y=3600.0) -> (x/y=w16:dbl)
  "WH/m3" <- w16
  n45 = Divide(x=w22, y=3600.0) -> (x/y=→"WH/Kg":dbl)
  n46 = Divide(x=w16, y=1000.0) -> (x/y=→"WH/Lit":dbl)
  n47 = Divide(x="Max V_out", y=w135) -> (x/y=→"Rf for Max i;  R+ C (EDL+Funct+ Analyte)":dbl)
  n48 = Divide(x="Max V_out", y=w131) -> (x/y=→"Rf for Max i;  R+ C (EDL+Funct)":dbl)
  n49 = Multiply(x="Energy Density  WH/Lit", y=1000.0) -> (x*y=w4:dbl)
  "Energy Density  WH/m3" <- w4
  n50 = Multiply(x=w4, y=w5) -> (x*y=w3:dbl)
  "Energy (wh/m3) / 1 NS pari with gap" <- w3
  n51 = Multiply(x=3600.0, y=w3) -> (x*y=→"J in 1 NS pair with gap":dbl)
  "Heat Generated (Energy) by Current in Metal films" <- "Energy (Heat; I^2R)"
  "CNT Thickness (CNT Length)" <- "Length of CNTs"
  "m-nm CNT" <- "m-nm l"
  "m-nm Dielectric" <- "Gap n-m"
  "um in 1 inch" <- w102
